vi "pcfs_acquire_stream.vi"(8 "error in (no error)":errorcluster, 11 "pcfs in":refnum<class "pcfs.lvclass">) -> (0 "error out":errorcluster, 3 "pcfs out":refnum<class "pcfs.lvclass">)   [LabVIEW 2015, in "pcfs.lvclass"]
uses:
  pcfs.lvclass
  pcfs.lvclass/pcfs.ctl
  Detector_Class/Picoquant/Picoquant_generic/picoquant_generic.lvclass
panel:
  in  "position_number":i32
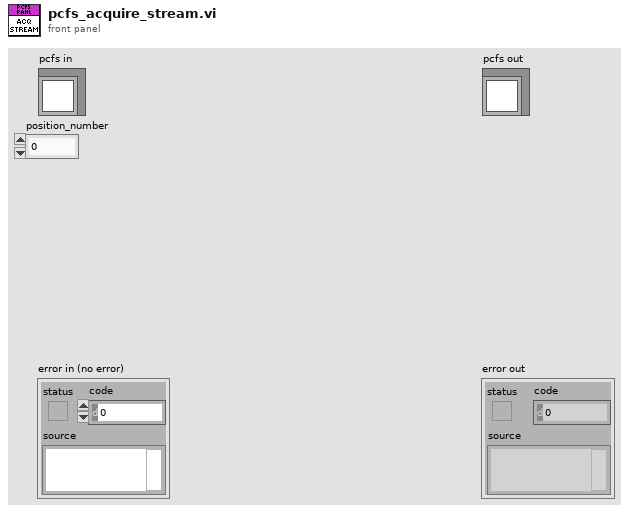
[diagram p1: front panel]
types:
  T1 = typedef "Rendezvous RefNum" = refnum<k1>
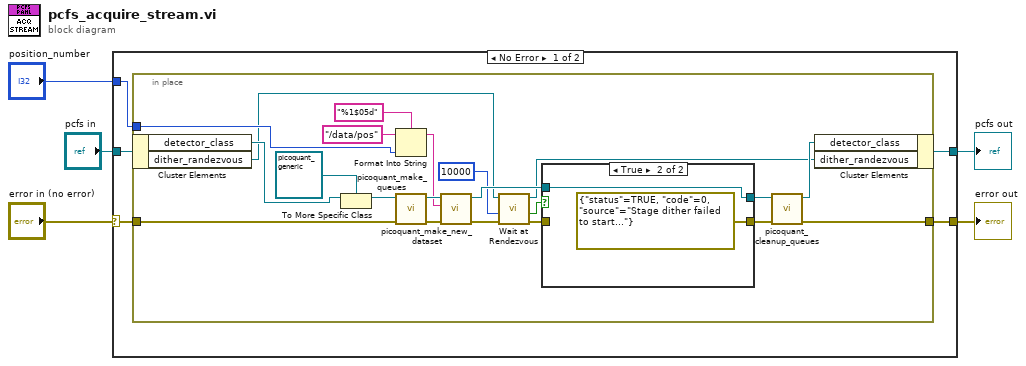
[diagram p0: block diagram]
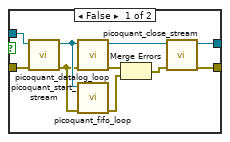
[diagram p2: hidden frame]
diagram:
  n1 = case shown="No Error" "error in (no error)" {
    selector: "error in (no error)" -> [w10 w45]
    tunnel: [w7 w45] -> w4
    tunnel: [w6 w44] -> w2
    tunnel: "pcfs in" -> [w9 w44]
    tunnel: "position_number" -> [w8 _]
    frame No Error {
      n2 = in-place {
        in-place-border: w10 -> [w24]
        in-place-border: w8 -> [w29]
        in-place-border: [w17] -> w7
        n3 = in-place-cluster #1(w9) -> ("detector_class"=w28:refnum<class "detector.lvclass">, "dither_randezvous"=w15:T1)
        n4 = To More Specific Class(target class=refnum<class "picoquant_generic.lvclass"> refnum ("picoquant_generic in"), reference=w28) -> (specific class reference=w23:refnum<class "picoquant_generic.lvclass">)  [unwired: 1 in, 1 out]
        n5 = Format Into String(format string="%1$05d", initial string="/data/pos" ("Path"), w29) -> (resulting string=w19:string)  [unwired: 1 in, 1 out]
        n6 = call "picoquant_make_queues.vi"("error in (no error)"=w24, "picoquant_generic in"=w23) -> ("error out"=w20:errorcluster, "picoquant_generic out"=w22:refnum<class "picoquant_generic.lvclass">)  [unwired: 8 in]
        n7 = call-dynamic "picoquant_make_new_dataset.vi"("error in (no error)"=w20, "dataset_path"=w19, "picoquant_generic in"=w22) -> ("error out"=w16:errorcluster, "picoquant_generic out"=w21:refnum<class "picoquant_generic.lvclass">)  [unwired: 7 in]
        n8 = call <vilib>:"Wait at Rendezvous.vi"("error in (no error)"=w16, "ms timeout (-1)"=10000, "rendezvous"=w15) -> ("error out"=w11:errorcluster, "timed out"=w12:bool, "rendezvous out"=w13:T1)  [unwired: 2 in]
        n9 = case shown="True" w12 {
          tunnel: [w35 w43] -> w26
          tunnel: [w34 errorcluster {"status"=TRUE, "code"=0, "source"="Stage dither failed to start..."} ("error out")] -> w25
          tunnel: w21 -> [w33 w43]
          tunnel: w11 -> [w32 _]
          frame False {
            n10 = call-dynamic "picoquant_start_stream.vi"("error in (no error)"=w32, "picoquant_generic in"=w33) -> ("error out"=w40:errorcluster, "picoquant_generic out"=w41:refnum<class "picoquant_generic.lvclass">)  [unwired: 8 in]
            n11 = call "picoquant_datalog_loop.vi"("error in (no error)"=w40, "picoquant_generic in"=w41) -> ("error out"=w39:errorcluster, "picoquant_generic out"=w37:refnum<class "picoquant_generic.lvclass">)  [unwired: 8 in]
            n12 = call "picoquant_fifo_loop.vi"("error in (no error)"=w40, "picoquant_generic in"=w41) -> ("error out"=w38:errorcluster)  [unwired: 8 in, 1 out]
            n13 = Merge Errors(w39, w38) -> (w36:errorcluster)
            n14 = call-dynamic "picoquant_close_stream.vi"("error in (no error)"=w36, "picoquant_generic in"=w37) -> ("error out"=w34:errorcluster, "picoquant_generic out"=w35:refnum<class "picoquant_generic.lvclass">)  [unwired: 8 in]
          }
          frame True {
          }
        }
        n15 = call "picoquant_cleanup_queues.vi"("error in (no error)"=w25, "picoquant_generic in"=w26) -> ("error out"=w17:errorcluster, "picoquant_generic out"=w18:refnum<class "picoquant_generic.lvclass">)  [unwired: 8 in]
        n16 = in-place-cluster #1("detector_class"=w18, "dither_randezvous"=w13) -> (w6:refnum<class "pcfs.lvclass">)
      }
    }
    frame Error {
    }
  }
  "error out" <- w4
  "pcfs out" <- w2
